vi "GetIndexRing—RhomSpiral.vi"(7 "Index":u64) -> (4 "Values at index":i64[](array[numeric]), 6 "Next vector #":u8, 8 "Current ring":i64, 10 "Ring size":i64, 15 "Ring position":u64)   [LabVIEW 2020]
panel:
  in  "file path (dialog if empty)":path=path "C:/Users/Lexa/DevProjects/Prometheus/Scalable packed voxel mapping/LookupTable-Rhombohedral.csv"
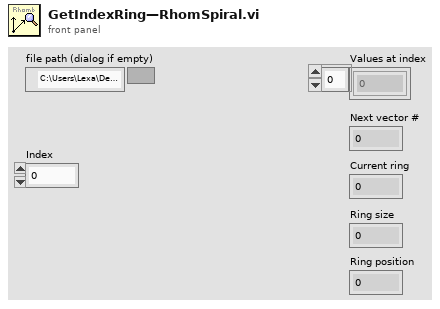
[diagram p1: front panel]
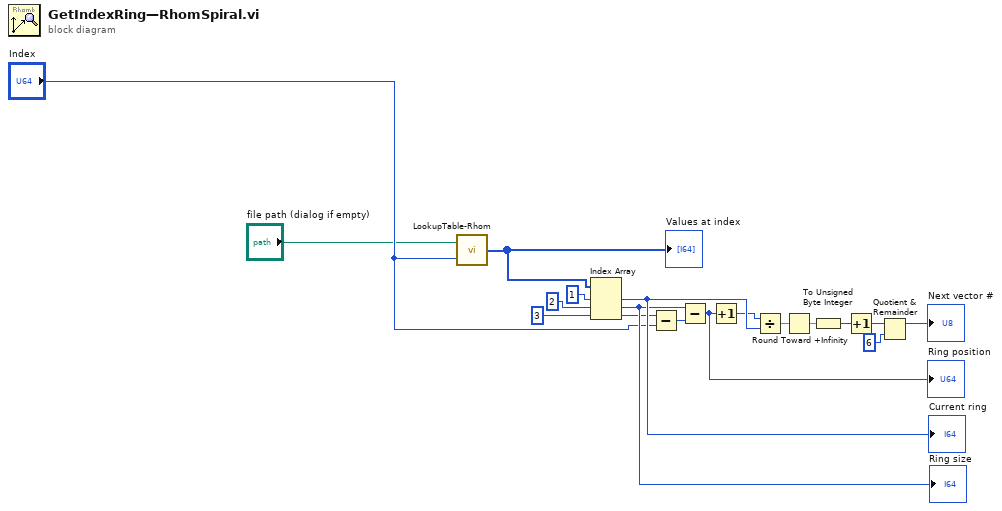
[diagram p0: block diagram]
diagram:
  n1 = call "LookupTable-Rhom.vi"("Lookup index"="Index", "file path (dialog if empty)"="file path (dialog if empty)") -> ("subarray"=w4:i64[])
  "Values at index" <- w4
  n2 = Index Array "Index Array"(array=w4, index #1=1 ("index"), index #2=2 ("index"), index #3=3 ("index")) -> (element #1=w17:i64, element #2=w16:i64, element #3=w8:i64)
  "Current ring" <- w17
  "Ring size" <- w16
  n3 = Subtract(x=w8, y="Index") -> (x-y=w7:u64)
  n4 = Subtract(x=w16, y=w7) -> (x-y=w18:u64)
  "Ring position" <- w18
  n5 = Increment(x=w18) -> (x+1=w11:u64)
  n6 = Divide(x=w11, y=w17) -> (x/y=w12:ext)
  n7 = Round Toward +Infinity(x=w12) -> (ceil(x): smallest int >= x=w13:ext)
  n8 = To Unsigned Byte Integer(number=w13) -> (unsigned 8bit integer=w14:u8)
  n9 = Increment(x=w14) -> (x+1=w15:u8)
  n10 = Quotient & Remainder(x=w15, y=u8 6) -> (x-y*floor(x/y)=→"Next vector #":u8)  [unwired: 1 out]
